vi "Control Panel No Objects.vi"(8 "error in (no error)":errorcluster) -> (0 "error out":errorcluster)   [LabVIEW 2009]
uses:
  Global/GPIB Numbers.vi
panel:
  in  "Step Rate Set":dbl=2000.0 min=32.0 max=3000.0 step=1.0
  out "Step Rate":ext
  in  "Set Step Rate":bool
  in  "Combined Position Set":dbl[unit] format="%#_8g"
  in  "Go to combined position\n(minimizing fine axis)":bool
  in  "Go to fine position":bool
  in  "Read to Control":bool
  in  "Fine Axis Set (um)":dbl[unit]
  in  "Coarse Axis Set (um)":dbl[unit]
  out "Combined Position (um)":ext[unit] format="%#_8g"
  out "Coarse Axis (um)":ext[unit]
  out "Fine Axis (um)":ext[unit]
  in  "Go to coarse position":bool
  in  "Read Positions":bool
  out "fine axis (steps)":dbl
  out "coarse axis(steps)":dbl
  in  "Calibrate Zero Positions":bool
  in  "stop":bool
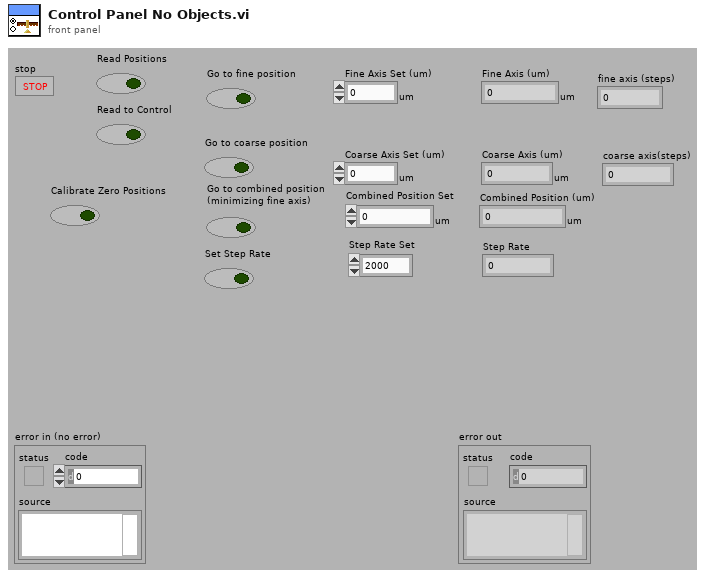
[diagram p1: front panel]
types:
  T1 = typedef "GPIB Type Def.ctl" = cluster{"Name":string, "bus":dbl, "GPIB":dbl, "GPIB as string":string, "byte":i32, "VISA Resource Name":refnum<visa-resource-name>}
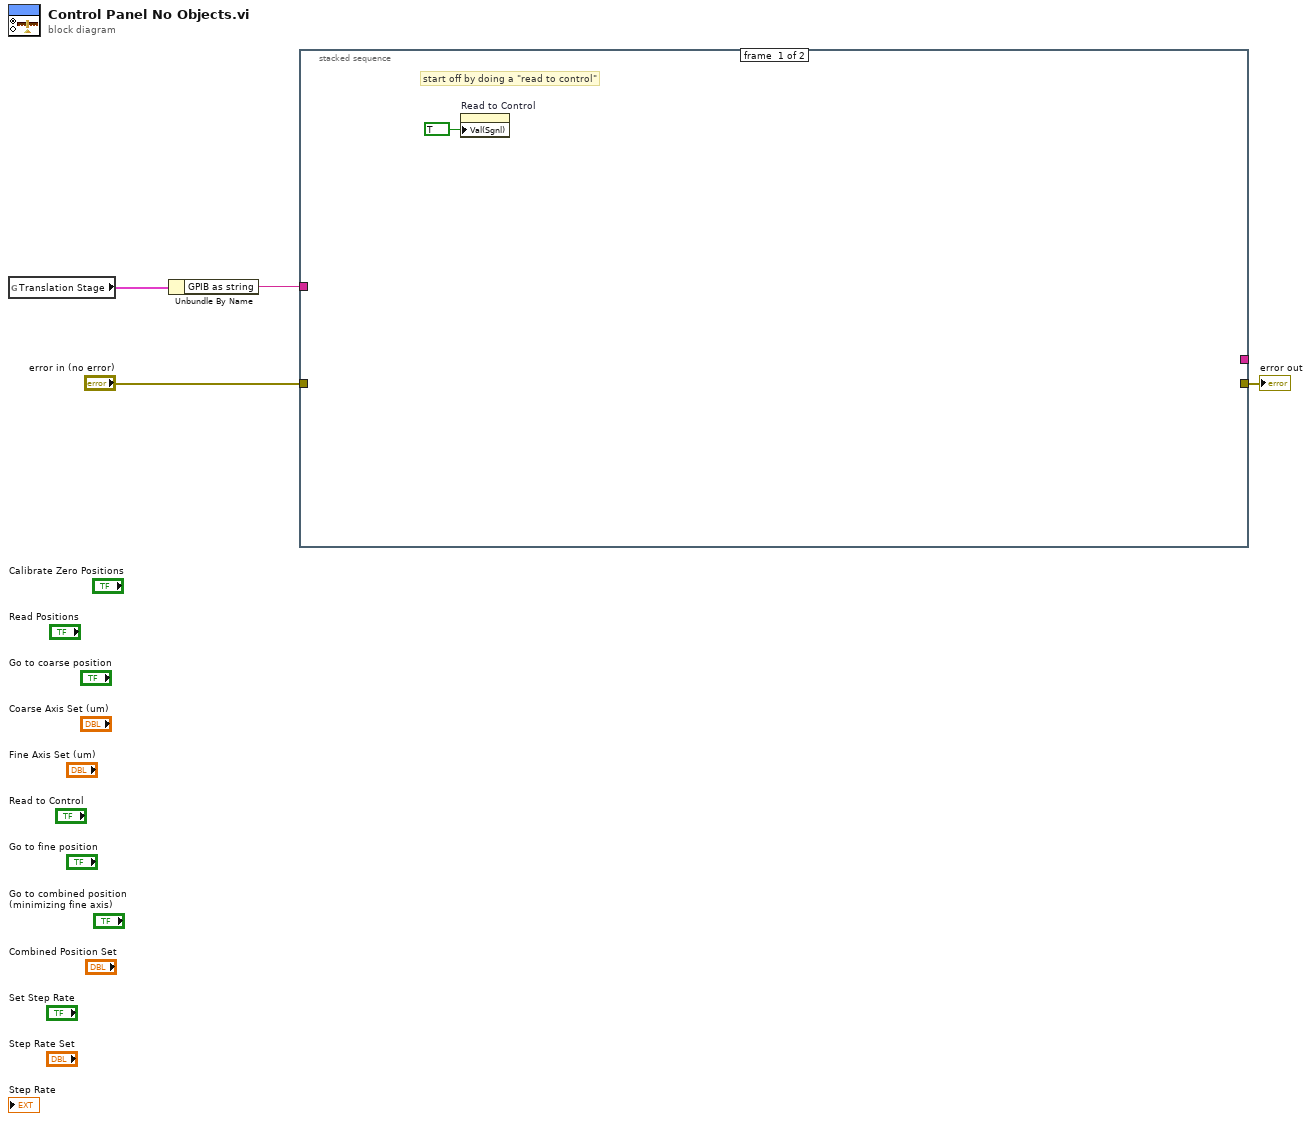
[diagram p0: block diagram]
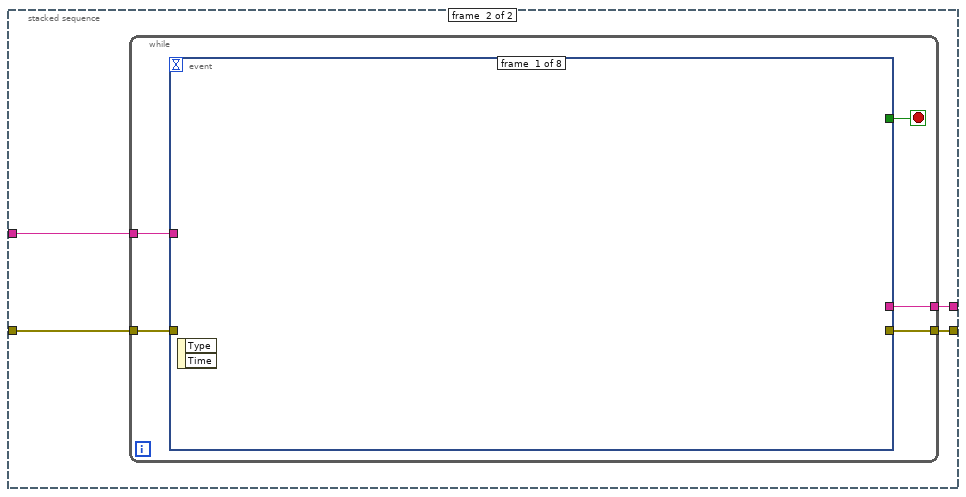
[diagram p2: hidden frame]
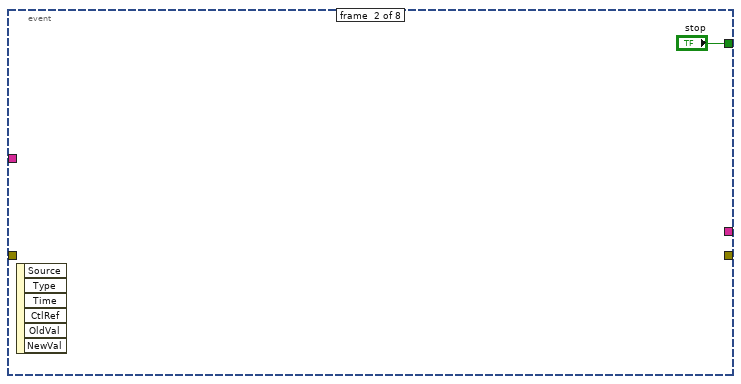
[diagram p3: hidden frame]
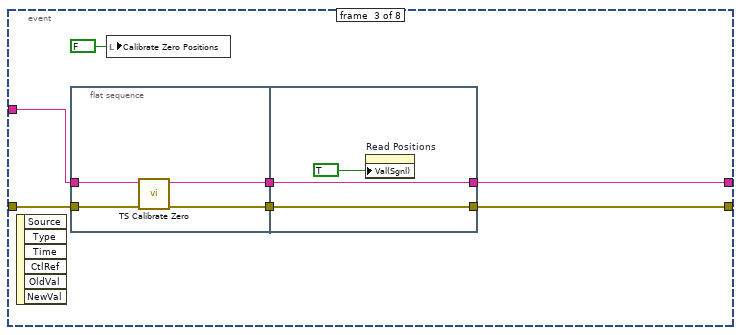
[diagram p4: hidden frame]
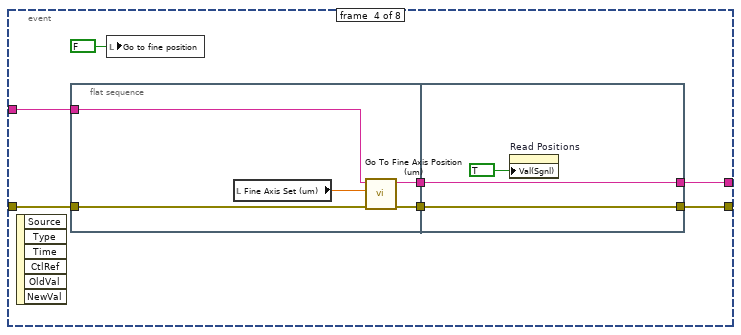
[diagram p5: hidden frame]
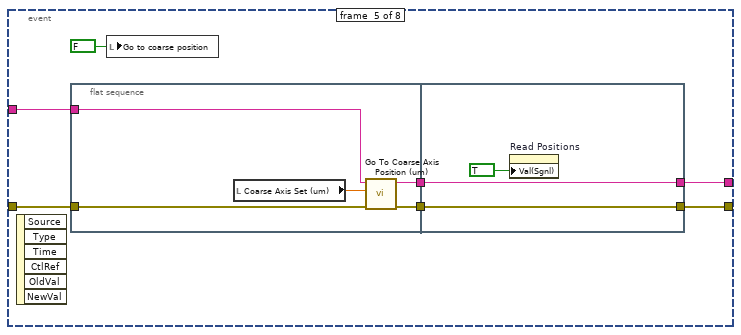
[diagram p6: hidden frame]
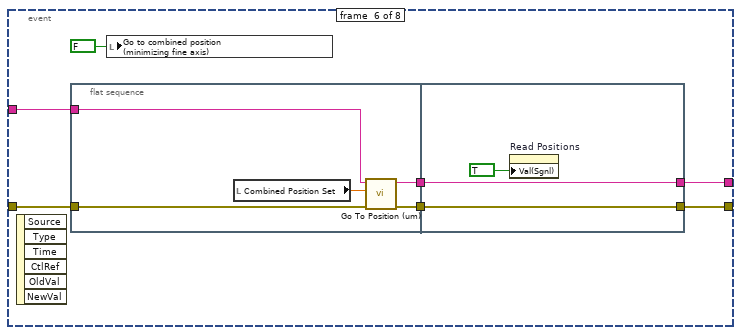
[diagram p7: hidden frame]
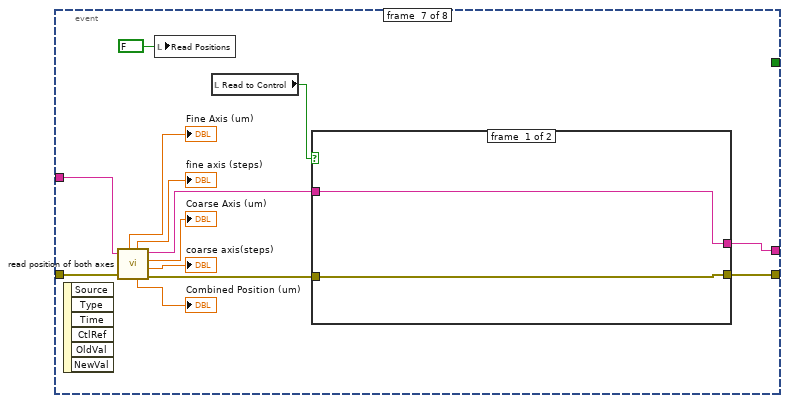
[diagram p8: hidden frame]
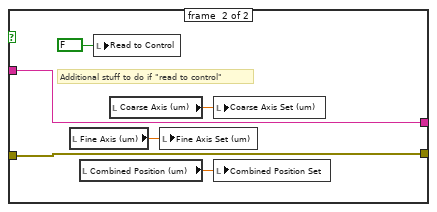
[diagram p9: hidden frame]
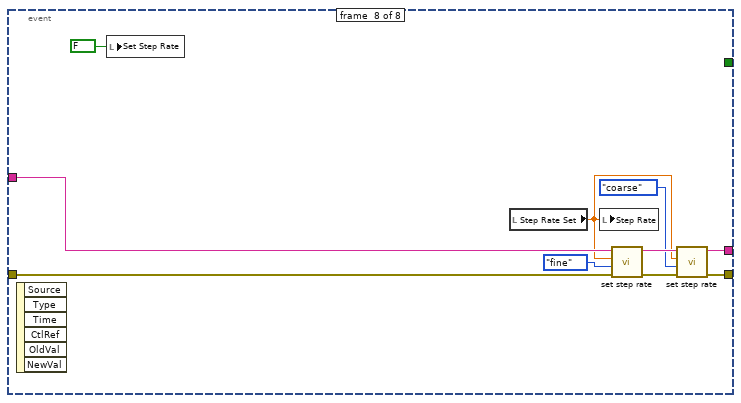
[diagram p10: hidden frame]
diagram:
  n1 = global read "GPIB Numbers.vi" "Translation Stage"() -> (w3:T1)
  n2 = Unbundle By Name(w3) -> ("GPIB as string"=w2:string)
  n3 = stacked-sequence {
    tunnel: "error in (no error)" -> [_ w9]
    tunnel: [_ w8] -> w4
    tunnel: w2 -> [_ w7]
    tunnel: [_ w6] -> _
    frame #0 {
      # "start off by doing a \"read to control\""
      n4 = property on="Read to Control" class="Bool (strict)"("Val(Sgnl)"=TRUE ("Value (Signaling)")) -> ()  [unwired: 2 in, 2 out]
    }
    frame #1 {
      n5 = while {
        tunnel: w9 -> [w13]
        tunnel: [w12] -> w8
        tunnel: w7 -> [w11]
        tunnel: [w10] -> w6
        stop <- w14 stop-if-true
        n6 = event shown="[7] \"Set Step Rate\": Value Change" {
          selector: _ -> [_ _ _ _ _ _ _ _]
          dyn-events: _ -> [_ _ _ _ _ _ _ _]
          timeout: _ -> [_ _ _ _ _ _ _ _]
          tunnel: [_ "stop" _ _ _ _ _ _] -> w14
          tunnel: w13 -> [_ _ w18 w33 w48 w63 w86 w104]
          tunnel: [_ _ w21 w35 w49 w64 w80 w98] -> w12
          tunnel: w11 -> [_ _ w19 w32 w45 w62 w79 w105]
          tunnel: [_ _ w20 w30 w47 w60 w75 w99] -> w10
          event #0 {
            n7 = event-data() -> ()  [unwired: 3 out]
          }
          event #1 {
            n8 = event-data() -> ()  [unwired: 7 out]
          }
          event #2 {
            n9 = event-data() -> ()  [unwired: 7 out]
            n10 = flat-sequence {
              tunnel: w19 -> [w26]
              tunnel: w18 -> [w25]
              tunnel: [w24] -> w17
              tunnel: [w23] -> w16
              tunnel: [w27] -> w21
              tunnel: [w28] -> w20
              tunnel: w17 -> [w28]
              tunnel: w16 -> [w27]
              frame #0 {
                n11 = call "TS Calibrate Zero.vi"("error out"=w25, "GPIB as string"=w26) -> ("error out 2"=w23:errorcluster, "GPIB # (out)"=w24:string)  [unwired: 8 out]
              }
              frame #1 {
                n12 = property on="Read Positions" class="Bool (strict)"("Val(Sgnl)"=TRUE ("Value (Signaling)")) -> ()  [unwired: 2 in, 2 out]
              }
            }
            n13 = local write "Calibrate Zero Positions"(FALSE ("Calibrate Zero Position")) -> ()
          }
          event #3 {
            n14 = event-data() -> ()  [unwired: 7 out]
            n15 = flat-sequence {
              tunnel: [w40] -> w34
              tunnel: w33 -> [w39]
              tunnel: w32 -> [w38]
              tunnel: [w37] -> w31
              tunnel: [w43] -> w35
              tunnel: w34 -> [w43]
              tunnel: w31 -> [w42]
              tunnel: [w42] -> w30
              frame #0 {
                n16 = local read "Fine Axis Set (um)"() -> (w41:dbl[unit])
                n17 = call "Go To Fine Axis Position (um).vi"("error in"=w39, "Fine Axis Position (um)"=w41, "GPIB # (in): def. 6"=w38) -> ("error out"=w40:errorcluster, "GPIB # (out)"=w37:string)  [unwired: 7 out]
              }
              frame #1 {
                n18 = property on="Read Positions" class="Bool (strict)"("Val(Sgnl)"=TRUE ("Value (Signaling)")) -> ()  [unwired: 2 in, 2 out]
              }
            }
            n19 = local write "Go to fine position"(FALSE ("Go to fine position")) -> ()
          }
          event #4 {
            n20 = event-data() -> ()  [unwired: 7 out]
            n21 = flat-sequence {
              tunnel: [w54] -> w51
              tunnel: w48 -> [w55]
              tunnel: [w53] -> w46
              tunnel: w45 -> [w52]
              tunnel: [w58] -> w49
              tunnel: w51 -> [w58]
              tunnel: [w57] -> w47
              tunnel: w46 -> [w57]
              frame #0 {
                n22 = local read "Coarse Axis Set (um)"() -> (w56:dbl[unit])
                n23 = call "Go To Coarse Axis Position (um).vi"("error in (no error)"=w55, "Coarse Axis Position (um)"=w56, "GPIB # (in): def. 6"=w52) -> ("error out"=w54:errorcluster, "GPIB # (out)"=w53:string)  [unwired: 7 out]
              }
              frame #1 {
                n24 = property on="Read Positions" class="Bool (strict)"("Val(Sgnl)"=TRUE ("Value (Signaling)")) -> ()  [unwired: 2 in, 2 out]
              }
            }
            n25 = local write "Go to coarse position"(FALSE ("Go to fine position")) -> ()
          }
          event #5 {
            n26 = event-data() -> ()  [unwired: 7 out]
            n27 = flat-sequence {
              tunnel: [w69] -> w66
              tunnel: w63 -> [w70]
              tunnel: w62 -> [w68]
              tunnel: [w67] -> w61
              tunnel: [w73] -> w64
              tunnel: w66 -> [w73]
              tunnel: [w72] -> w60
              tunnel: w61 -> [w72]
              frame #0 {
                n28 = local read "Combined Position Set"() -> (w71:dbl[unit])
                n29 = call "Go To Position (um).vi"("error in (no error)"=w70, "Position (um)"=w71, "GPIB # (in): def. 6"=w68) -> ("error out"=w69:errorcluster, "GPIB # (out)"=w67:string)  [unwired: 7 out]
              }
              frame #1 {
                n30 = property on="Read Positions" class="Bool (strict)"("Val(Sgnl)"=TRUE ("Value (Signaling)")) -> ()  [unwired: 2 in, 2 out]
              }
            }
            n31 = local write "Go to combined position\n(minimizing fine axis)"(FALSE ("Go to fine position")) -> ()
          }
          event #6 {
            n32 = event-data() -> ()  [unwired: 7 out]
            n33 = call "read position of both axes.vi"("GPIB # (in): def. 6"=w79, "error in (no error)"=w86) -> ("fine axis (um)"=→"Fine Axis (um)":ext[unit], "fine axis (steps)"=→"fine axis (steps)":dbl, "GPIB # (out)"=w76:string, "coarse axis (um)"=→"Coarse Axis (um)":ext[unit], "combined position (um)"=→"Combined Position (um)":ext[unit], "coarse axis(steps)"=→"coarse axis(steps)":dbl, "error out"=w81:errorcluster)  [unwired: 2 out]
            n34 = local write "Read Positions"(FALSE ("Read Positions")) -> ()
            n35 = local read "Read to Control"() -> (w82:bool)
            n36 = case shown="True" w82 {
              tunnel: w81 -> [w89 w91]
              tunnel: [w89 w91] -> w80
              tunnel: w76 -> [w88 w90]
              tunnel: [w88 w90] -> w75
              frame #0 {
              }
              frame #1 {
                # "Additional stuff to do if \"read to control\""
                n37 = local read "Fine Axis (um)"() -> (w93:ext[unit])
                n38 = local read "Combined Position (um)"() -> (w92:ext[unit])
                n39 = local write "Read to Control"(FALSE ("Read Positions")) -> ()
                n40 = local read "Coarse Axis (um)"() -> (w94:ext[unit])
                n41 = local write "Fine Axis Set (um)"(w93) -> ()
                n42 = local write "Coarse Axis Set (um)"(w94) -> ()
                n43 = local write "Combined Position Set"(w92) -> ()
              }
            }
          }
          event #7 {
            n44 = event-data() -> ()  [unwired: 7 out]
            n45 = local write "Set Step Rate"(FALSE) -> ()
            n46 = local read "Step Rate Set"() -> (w96:dbl)
            n47 = local write "Step Rate"(w96) -> ()
            n48 = call "set step rate.vi"("error in"=w104, "axis (def: fine)"=enum16{"fine", "coarse"}."fine", "step rate"=w96, "GPIB # (in): def. 6"=w105) -> ("error out"=w101:errorcluster, "GPIB # (out)"=w102:string)  [unwired: 6 out]
            n49 = call "set step rate.vi"("error in"=w101, "axis (def: fine)"=enum16{"fine", "coarse"}."coarse", "step rate"=w96, "GPIB # (in): def. 6"=w102) -> ("error out"=w98:errorcluster, "GPIB # (out)"=w99:string)  [unwired: 6 out]
          }
        }
      }
    }
  }
  "error out" <- w4
